vi "Variant to JSON String.vi"(0 "Variant in":variant, 7 "enable LabVIEW extensions? (T)":bool=TRUE, 9 "pretty print? (F)":bool, 11 "error in (no error)":errorcluster) -> (4 "Variant out":variant, 8 "String":string, 15 "error out":errorcluster)   [LabVIEW 2017, in "Advanced Variant Tools.lvlib"]
uses:
  Advanced Variant Tools.lvlib
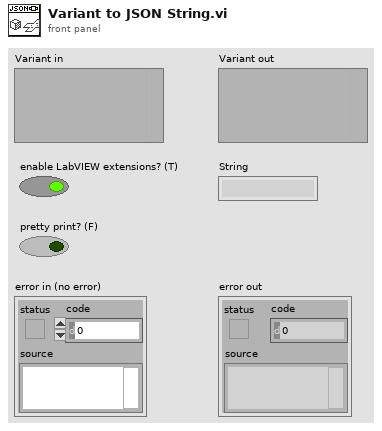
[diagram p1: front panel]
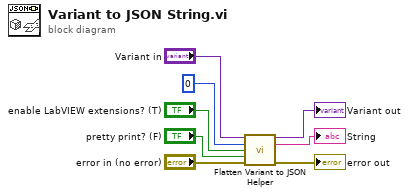
[diagram p0: block diagram]
diagram:
  n1 = call "Flatten Variant to JSON Helper.vi"("Variant in"="Variant in", "indent"=0, "enable LabVIEW extensions? (T)"="enable LabVIEW extensions? (T)", "pretty print? (T)"="pretty print? (F)", "error in (no error)"="error in (no error)") -> ("Variant out"=→"Variant out":variant, "String"=→"String":string, "error out"=→"error out":errorcluster)  [unwired: 8 in]
